vi "Write Search Path.vi"(8 "Error In":errorcluster, 10 "Search Path":path[](array[path]), 11 "File In":refnum<class "File.lvclass">) -> (0 "Error Out":errorcluster, 3 "File Out":refnum<class "File.lvclass">)   [LabVIEW 2018, in "Toolkit.lvlib" / "Loaders.lvlib" / "File.lvclass"]
doc: "Sets the search path used to locate partial Mustache template files if the <B>Root</B> is empty or <Not a Path>.\n\n<B>File In/Out</B> - Represents a file partial loader, where partial Mustache templates are loaded from files.\n\n<B>Search Path</B> - An array of folder paths that are used to find a partial Mustache template stored on disk. The file stem (file name without extension) is the partial tag's key."
uses:
  File.lvclass
  File.lvclass/File.ctl
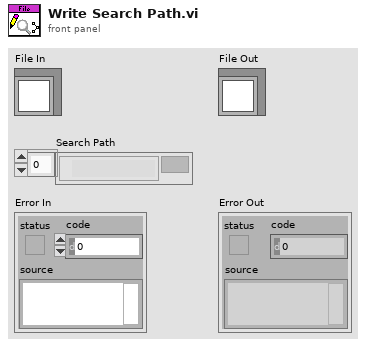
[diagram p1: front panel]
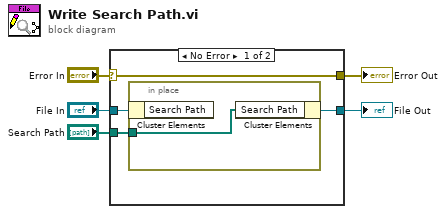
[diagram p0: block diagram]
diagram:
  n1 = case shown="No Error" "Error In" {
    selector: "Error In" -> [w9 w11]
    tunnel: [w9 w11] -> w4
    tunnel: [w6 w12] -> w2
    tunnel: "File In" -> [w8 w12]
    tunnel: "Search Path" -> [w7 _]
    frame No Error {
      n2 = in-place {
        in-place-border: w7 -> [w10]
        n3 = in-place-cluster #1(w8) -> ()  [unwired: 1 out]
        n4 = in-place-cluster #1("Search Path"=w10) -> (w6:refnum<class "File.lvclass">)
      }
    }
    frame Error {
    }
  }
  "Error Out" <- w4
  "File Out" <- w2
